vi "Read tx transfer settings.vi"(8 "error in (no error)":errorcluster, 11 "UDPlog Transfer Tx Configuration in":refnum<class "UDPlog Transfer Tx Configuration.lvclass">) -> (0 "error out":errorcluster, 2 "tx transfer settings":T1, 3 "UDPlog Transfer Tx Configuration out":refnum<class "UDPlog Transfer Tx Configuration.lvclass">)   [LabVIEW 2023, in "UDPlog.lvlib" / "UDPlog Transfer Tx Configuration.lvclass"]
uses:
  UDPlog Transfer Tx Configuration.lvclass
  UDPlog Transfer Tx Configuration.lvclass/UDPlog Transfer Tx Configuration.ctl
  Tx Transfer Settings.ctl
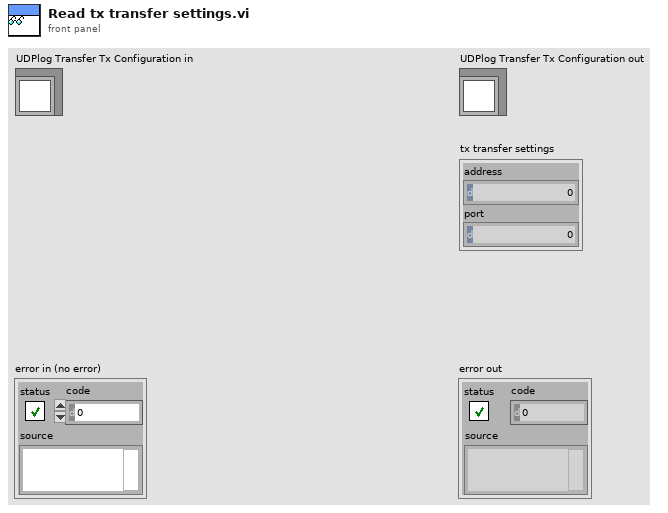
[diagram p1: front panel]
types:
  T1 = typedef "Tx Transfer Settings.ctl" = cluster{"address":u32, "port":u16}
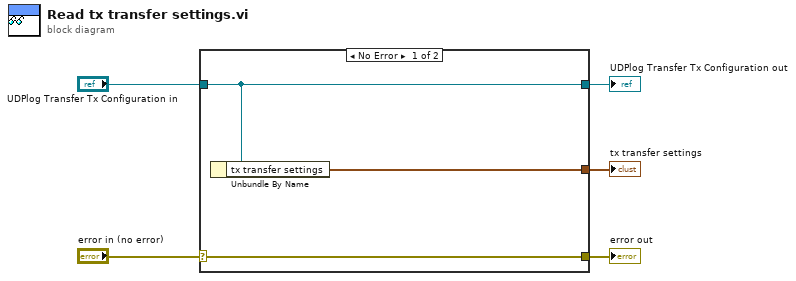
[diagram p0: block diagram]
diagram:
  n1 = case shown="No Error" "error in (no error)" {
    selector: "error in (no error)" -> [w8 w9]
    tunnel: [w8 w9] -> w4
    tunnel: [w7 w10] -> w2
    tunnel: "UDPlog Transfer Tx Configuration in" -> [w7 w10]
    tunnel: [w6 _] -> w1
    frame No Error {
      n2 = Unbundle By Name(w7) -> ("tx transfer settings"=w6:T1)
    }
    frame Error {
    }
  }
  "error out" <- w4
  "UDPlog Transfer Tx Configuration out" <- w2
  "tx transfer settings" <- w1
